vi "SUB-FTS_Result_divide.vi"(10 "Table Value":string[][](array[string]), 11 "Test profile":string[][](array[string])=[["Load(1)-0lb", "0", "1000", "0", "0"], ["Init(1)-70lb", "70", "1000", "0", "0"], ["Init(2)-140lb", "140", "1000", "0", "0"], ["Init(1)-70lb", "70", "1000", "0", "0"], ["Init(2)-140lb", "140", "1000", "0", "0"], ["Load(1)-0lb", "0", "10000", "1", "1"], ["Load(2)-10lb", "10", "3000", "0", "1"], ["Load(3)-20lb", "20", "3000", "0", "1"], ["Load(4)-40lb", "40", "3000", "0", "1"], ["Load(5)-60lb", "60", "3000", "0", "1"], ["Load(6)-80lb", "80", "3000", "0", "1"]]) -> (2 "Load Test data":string[][](array[string]), 3 "Cal data":string[][](array[string]))   [LabVIEW 2015]
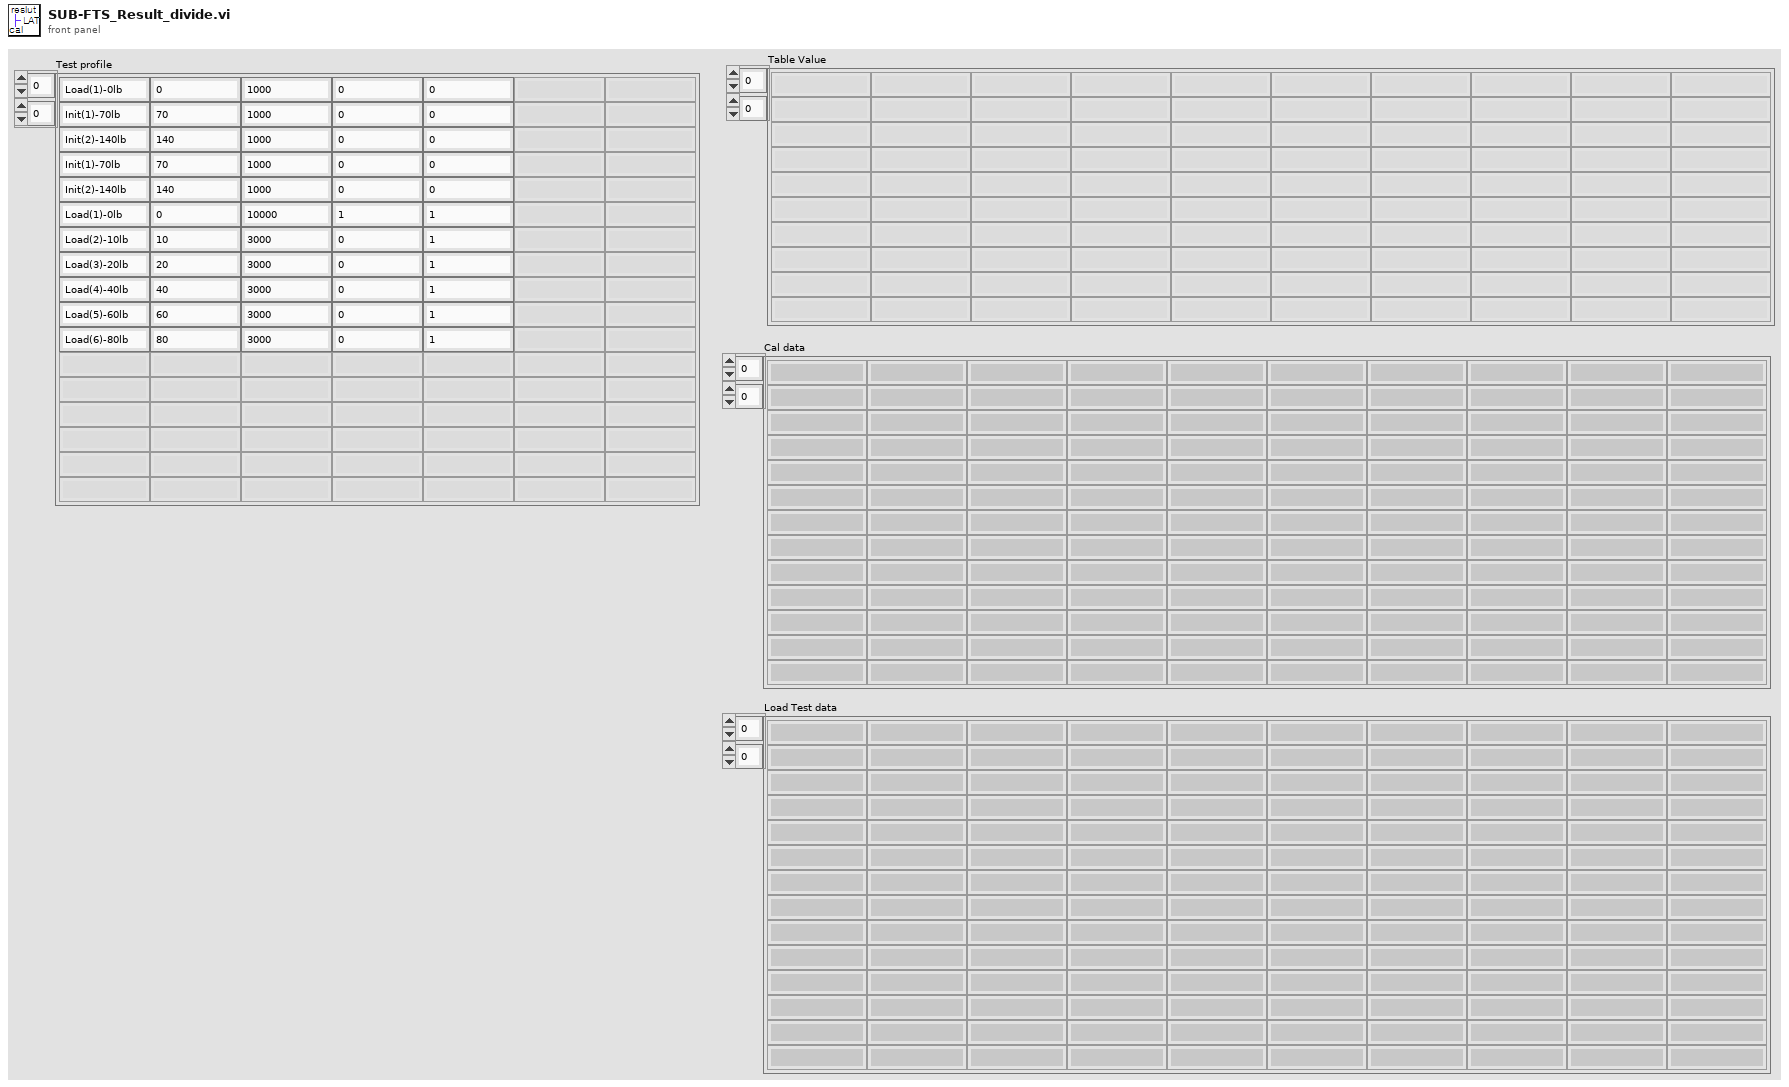
[diagram p1: front panel]
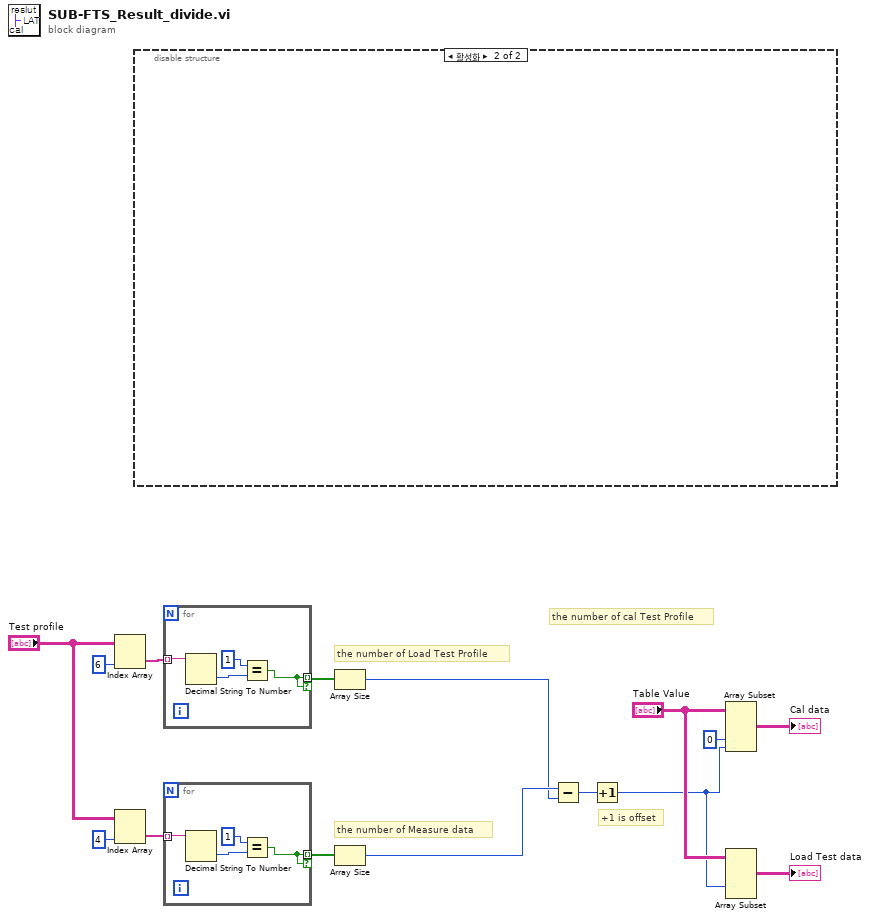
[diagram p0: block diagram]
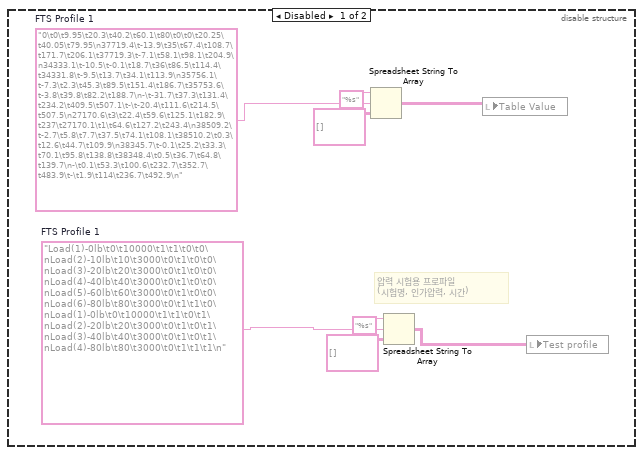
[diagram p2: hidden frame]
diagram:
  # "the number of cal Test Profile"
  # "the number of Measure data"
  # "+1 is offset"
  # "the number of Load Test Profile"
  n1 = Index Array(array="Test profile", index (col)=6 ("비활성화된 인덱스 (열)")) -> (element=w8:string[])  [unwired: 1 in]
  n2 = Index Array(array="Test profile", index (col)=4 ("비활성화된 인덱스 (열)")) -> (element=w5:string[])  [unwired: 1 in]
  n3 = disable-structure shown="활성화" {
    frame Disabled {
      w17 = "0\t0\t9.95\t20.3\t40.2\t60.1\t80\t0\t0\t20.25\t40.05\t79.95\n37719.4\t-13.9\t35\t67.4\t108.7\t171.7\t206.1\t37719.3\t-7.1\t58.1\t98.1\t204.9\n34333.1\t-10.5\t-0.1\t18.7\t36\t86.5\t114.4\t34331.8\t-9.5\t13.7\t34.1\t113.9\n35756.1\t-7.3\t2.3\t45.3\t89.5\t151.4\t186.7\t35753.6\t-3.8\t39.8\t82.2\t188.7\n-\t-31.7\t37.3\t131.4\t234.2\t409.5\t507.1\t-\t-20.4\t111.6\t214.5\t507.5\n27170.6\t3\t22.4\t59.6\t125.1\t182.9\t237\t27170.1\t1\t64.6\t127.2\t243.4\n38509.2\t-2.7\t5.8\t7.7\t37.5\t74.1\t108.1\t38510.2\t0.3\t12.6\t44.7\t109.9\n38345.7\t-0.1\t25.2\t33.3\t70.1\t95.8\t138.8\t38348.4\t0.5\t36.7\t64.8\t139.7\n-\t0.1\t53.3\t100.6\t232.7\t352.7\t483.9\t-\t1.9\t114\t236.7\t492.9\n"  # FTS Profile 1
      w21 = "Load(1)-0lb\t0\t10000\t1\t1\t0\t0\nLoad(2)-10lb\t10\t3000\t0\t1\t0\t0\nLoad(3)-20lb\t20\t3000\t0\t1\t0\t0\nLoad(4)-40lb\t40\t3000\t0\t1\t0\t0\nLoad(5)-60lb\t60\t3000\t0\t1\t0\t0\nLoad(6)-80lb\t80\t3000\t0\t1\t1\t0\nLoad(1)-0lb\t0\t10000\t1\t1\t0\t1\nLoad(2)-20lb\t20\t3000\t0\t1\t0\t1\nLoad(3)-40lb\t40\t3000\t0\t1\t0\t1\nLoad(4)-80lb\t80\t3000\t0\t1\t1\t1\n"  # FTS Profile 1
      # "압력 시험용 프로파일\n(시험명, 인가압력, 시간)"
      n4 = Spreadsheet String To Array(format string="%s" ("포맷 문자열"), spreadsheet string=w17, array type (2D Dbl)=string[][] [] ("배열 타입(2D Dbl)")) -> (array=w16:string[][])  [unwired: 1 in]
      n5 = Spreadsheet String To Array(format string="%s" ("포맷 문자열"), spreadsheet string=w21, array type (2D Dbl)=string[][] [] ("배열 타입(2D Dbl)")) -> (array=w20:string[][])  [unwired: 1 in]
      n6 = local write "Table Value"(w16) -> ()
      n7 = local write "Test profile"(w20) -> ()
    }
    frame Enabled {
    }
  }
  n8 = for {
    tunnel: w8 -> [w27] mode=indexing
    tunnel: [w24] -> w9 mode=indexing if=w24
    n9 = Decimal String To Number(string=w27) -> (number=w26:i32)  [unwired: 2 in, 1 out]
    n10 = Equal?(x=1, y=w26) -> (x = y?=w24:bool)
  }
  n11 = for {
    tunnel: w5 -> [w31] mode=indexing
    tunnel: [w28] -> w4 mode=indexing if=w28
    n12 = Decimal String To Number(string=w31) -> (number=w30:i32)  [unwired: 2 in, 1 out]
    n13 = Equal?(x=1, y=w30) -> (x = y?=w28:bool)
  }
  n14 = Array Size(array=w9) -> (size(s)=w2:i32)
  n15 = Array Size(array=w4) -> (size(s)=w3:i32)
  n16 = Subtract(x=w3, y=w2) -> (x-y=w1:i32)
  n17 = Increment(x=w1) -> (x+1=w10:i32)
  n18 = Array Subset(array="Table Value", index (col)=0 ("인덱스"), length (col)=w10) -> (→"Cal data":string[][])  [unwired: 2 in]
  n19 = Array Subset(array="Table Value", index (col)=w10) -> (→"Load Test data":string[][])  [unwired: 3 in]
